vi "Queue Nested Teardown.vi"(11 "Base Queue jettl in":refnum<class "Base Queue jettl.lvclass">) -> (3 "Base Queue jettl out":refnum<class "Base Queue jettl.lvclass">)   [LabVIEW 2021, in "jettl.lvlib" / "Base Queue jettl.lvlib" / "Base Queue jettl.lvclass"]
uses:
  Base Queue jettl.lvclass
  Msg Strategy/Teardown/Teardown Msg/Teardown Msg.lvclass
  C:/git/jettl/src/jettl/Msg/Msg/Msg.lvclass
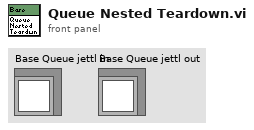
[diagram p1: front panel]
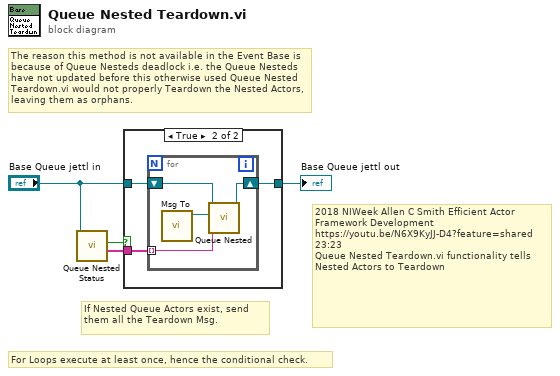
[diagram p0: block diagram]
diagram:
  # "2018 NIWeek Allen C Smith Efficient Actor Framework Development\nhttps://youtu.be/N6X9KyJJ-D4?feature=shared\n23:23\nQueue Nested Teardown.vi functionality tells Nested Actors to Teardown"
  # "For Loops execute at least once, hence the conditional check."
  # "If Nested Queue Actors exist, send them all the Teardown Msg."
  # "The reason this method is not available in the Event Base is because of Queue Nesteds deadlock i.e. the Queue Nesteds have not updated before this otherwise used Queue Nested Teardown.vi would not properly Teardown the Nested Actors, leaving them as orphans."
  n1 = call-dynamic "Queue Nested Status.vi"("Base Queue jettl in"="Base Queue jettl in") -> ("Queue Nested Aliases"=w3:string[], "Any Exist?"=w4:bool)  [unwired: 8 in, 1 out]
  n2 = case shown="True" w4 {
    tunnel: [w5 w8] -> w1
    tunnel: "Base Queue jettl in" -> [w5 w7]
    tunnel: w3 -> [_ w6]
    frame False {
    }
    frame True {
      n3 = for {
        tunnel: w6 -> [w11] mode=indexing
        shift-right: [w9] -> w8
        shift-left: w7 -> [w10]
        n4 = call "Msg To.vi"() -> ("Teardown Msg out"=w12:refnum<class "Teardown Msg.lvclass">)  [unwired: 11 in]
        n5 = call-dynamic "Queue Nested.vi"("Alias"=w11, "Msg Strategy"=w12, "Base Queue jettl in"=w10) -> ("Base Queue jettl out"=w9:refnum<class "Base Queue jettl.lvclass">)  [unwired: 8 in]
      }
    }
  }
  "Base Queue jettl out" <- w1
